vi "Functional Global - Control Configurations.vi"(7 "Functional Global Operation (Read)":T2=enum."Read" caption="功能全局操作（读取）", 11 "Control Configurations in":T1[](array[typedef]) caption="控制配置输入") -> (3 "Control Configurations out":T1[](array[typedef]) caption="控制配置输出")   [LabVIEW 2013]
uses:
  controls/Functional Global Operation.ctl
  controls/Control Configuration.ctl
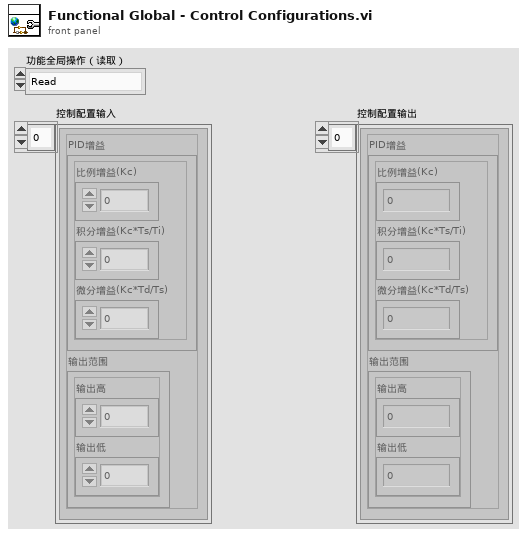
[diagram p1: front panel]
types:
  T1 = typedef "Control Configuration.ctl" = cluster{"PID Gains":cluster{"proportional gain (Kc)":dbl, "integral gain (Kc*Ts/Ti)":dbl, "derivative gain (Kc*Td/Ts)":dbl}, "Output Range":cluster{"output high":dbl, "output low":dbl}}
  T2 = typedef "Functional Global Operation.ctl" = enum16{"Initialize", "Read", "Write"}
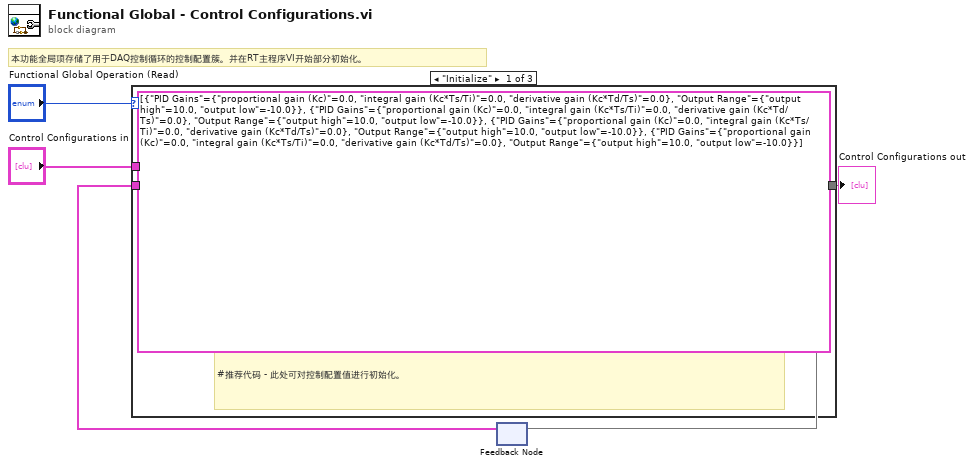
[diagram p0: block diagram]
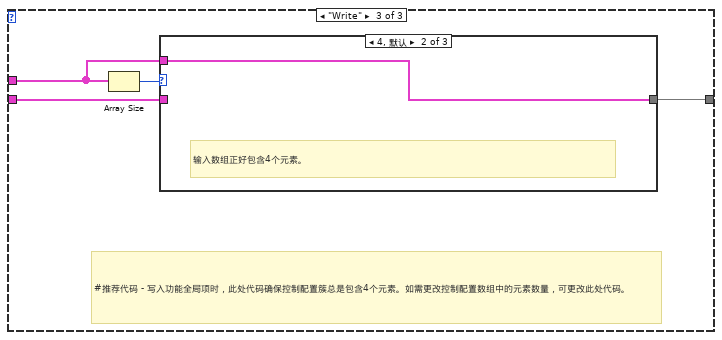
[diagram p3: hidden frame]
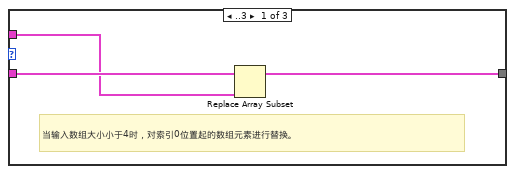
[diagram p4: hidden frame]
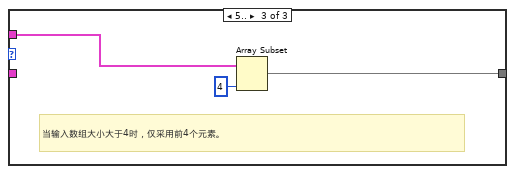
[diagram p5: hidden frame]
diagram:
  # "本功能全局项存储了用于DAQ控制循环的控制配置簇。并在RT主程序VI开始部分初始化。"
  n1 = feedback #1() -> (w1:T1[])  [unwired: 1 in]
  n2 = case shown="\"Initialize\"" "Functional Global Operation (Read)" {
    tunnel: "Control Configurations in" -> [_ _ w8]
    tunnel: [T1[] [{"PID Gains"={"proportional gain (Kc)"=0.0, "integral gain (Kc*Ts/Ti)"=0.0, "derivative gain (Kc*Td/Ts)"=0.0}, "Output Range"={"output high"=10.0, "output low"=-10.0}}, {"PID Gains"={"proportional gain (Kc)"=0.0, "integral gain (Kc*Ts/Ti)"=0.0, "derivative gain (Kc*Td/Ts)"=0.0}, "Output Range"={"output high"=10.0, "output low"=-10.0}}, {"PID Gains"={"proportional gain (Kc)"=0.0, "integral gain (Kc*Ts/Ti)"=0.0, "derivative gain (Kc*Td/Ts)"=0.0}, "Output Range"={"output high"=10.0, "output low"=-10.0}}, {"PID Gains"={"proportional gain (Kc)"=0.0, "integral gain (Kc*Ts/Ti)"=0.0, "derivative gain (Kc*Td/Ts)"=0.0}, "Output Range"={"output high"=10.0, "output low"=-10.0}}] ("Control Configurations in") w6 w7] -> w2
    tunnel: w1 -> [_ w6 w9]
    frame "Initialize" {
      # "#推荐代码 - 此处可对控制配置值进行初始化。"
    }
    frame "Read", Default {
    }
    frame "Write" {
      # "#推荐代码 - 写入功能全局项时，此处代码确保控制配置簇总是包含4个元素。如需更改控制配置数组中的元素数量，可更改此处代码。"
      n3 = Array Size(array=w8) -> (size(s)=w10:i32)
      n4 = case shown="4, 默认" w10 {
        tunnel: w9 -> [w13 _ _]
        tunnel: w8 -> [w12 w14 w17]
        tunnel: [w11 w14 w15] -> w7
        frame ..3 {
          # "当输入数组大小小于4时，对索引0位置起的数组元素进行替换。"
          n5 = Replace Array Subset(array=w13, new element=w12) -> (w11:T1[])  [unwired: 1 in]
        }
        frame 4, Default {
          # "输入数组正好包含4个元素。"
        }
        frame 5.. {
          # "当输入数组大小大于4时，仅采用前4个元素。"
          n6 = Array Subset(array=w17, length=4) -> (w15:T1[])  [unwired: 1 in]
        }
      }
    }
  }
  "Control Configurations out" <- w2
  n7 = feedback-in #1(w2) -> ()
